vi "ScriptAccessorVIs.vi"(5 "Virtual Folder Name":string, 6 "Create as Properties":bool, 7 "Include error terminals":bool, 8 "error in (no error)":errorcluster, 9 "Make Class Terminals Dynamic":bool, 10 "Access":T1, 11 "BaseAccessorScripter in":refnum<class "BaseAccessorScripter.lvclass">) -> (0 "error out":errorcluster, 3 "BaseAccessorScripter out":refnum<class "BaseAccessorScripter.lvclass">)   [LabVIEW 2021, in "MemberVICreation.lvlib" / "BaseAccessorScripter.lvclass"]
uses:
  <resource>/Framework/Providers/LVClassLibrary/NewAccessors/BaseAccessorScripter/BaseAccessorScripter.lvclass
  <resource>/Framework/Providers/LVClassLibrary/NewAccessors/CLSUIP_Access.ctl
  <resource>/Framework/Providers/LVClassLibrary/NewAccessors/BaseAccessorScripter/BaseAccessorScripter.lvclass/BaseAccessorScripter.ctl
  <resource>/Framework/Providers/LVClassLibrary/NewAccessors/MemberVICreation.lvlib
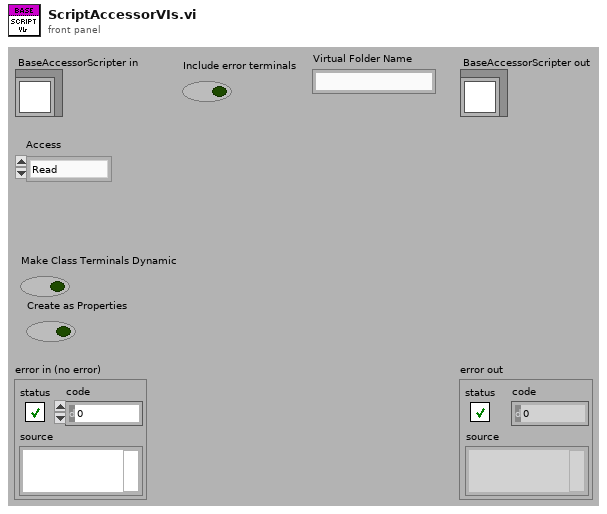
[diagram p1: front panel]
types:
  T1 = typedef "MemberVICreation.lvlib/CLSUIP_Access.ctl" = enum16{"Read", "Write", "R/W"}
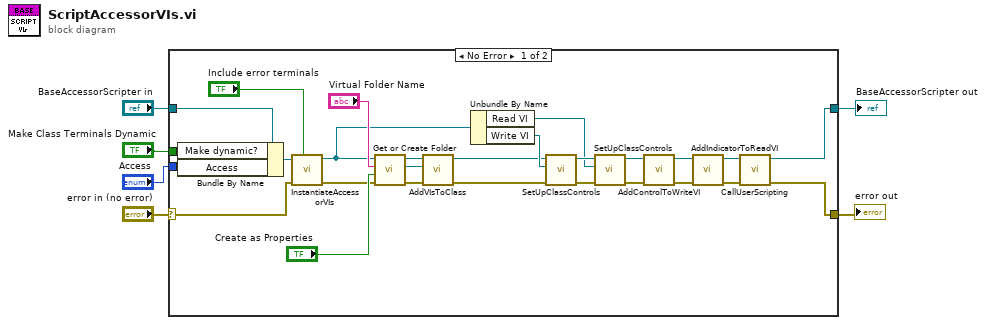
[diagram p0: block diagram]
diagram:
  n1 = case shown="No Error" "error in (no error)" {
    selector: "error in (no error)" -> [w29 w35]
    tunnel: [w19 w35] -> w5
    tunnel: [w18 w34] -> w3
    tunnel: "BaseAccessorScripter in" -> [w33 w34]
    tunnel: "Make Class Terminals Dynamic" -> [w32 _]
    tunnel: "Access" -> [w31 _]
    frame No Error {
      n2 = Bundle By Name(cluster=w33, "Make dynamic?"=w32, "Access"=w31) -> (w30:refnum<class "BaseAccessorScripter.lvclass">)
      n3 = call <resource>:"InstantiateAccessorVIs.vi"("Include error terminals"="Include error terminals", "error in (no error)"=w29, "BaseAccessorScripter in"=w30) -> ("error out"=w10:errorcluster, "BaseAccessorScripter out"=w7:refnum<class "BaseAccessorScripter.lvclass">)  [unwired: 7 out]
      n4 = call-dynamic "Get or Create Folder.vi"("error in (no error)"=w10, "CreateAsProperties"="Create as Properties", "Virtual Folder Name"="Virtual Folder Name", "BaseAccessorScripter in"=w7) -> ("error out"=w14:errorcluster, "Folder Refnum out"=w13:refnum<vi>, "BaseAccessorScripter out"=w17:refnum<class "BaseAccessorScripter.lvclass">)  [unwired: 5 in]
      n5 = call <resource>:"AddVIsToClass.vi"("error in (no error)"=w14, "Destination Folder"=w13, "BaseAccessorScripter in"=w17) -> ("error out"=w9:errorcluster, "BaseAccessorScripter out"=w8:refnum<class "BaseAccessorScripter.lvclass">)  [unwired: 7 in]
      n6 = Unbundle By Name(w7) -> ("Read VI"=w25:refnum<vi>, "Write VI"=w26:refnum<vi>)
      n7 = call <resource>:"SetUpClassControls.vi"("error in (no error)"=w9, "VI Reference"=w26, "Scripter Class"=w8) -> ("error out"=w27:errorcluster, "Scripter Class out"=w28:refnum<class "BaseAccessorScripter.lvclass">)  [unwired: 7 out]
      n8 = call <resource>:"SetUpClassControls.vi"("error in (no error)"=w27, "VI Reference"=w25, "Scripter Class"=w28) -> ("error out"=w23:errorcluster, "Scripter Class out"=w24:refnum<class "BaseAccessorScripter.lvclass">)  [unwired: 7 out]
      n9 = call <resource>:"AddControlToWriteVI.vi"("error in (no error)"=w23, "BaseAccessorScripter in"=w24) -> ("error out"=w21:errorcluster, "BaseAccessorScripter out"=w22:refnum<class "BaseAccessorScripter.lvclass">)  [unwired: 8 out]
      n10 = call <resource>:"AddIndicatorToReadVI.vi"("error in (no error)"=w21, "BaseAccessorScripter in"=w22) -> ("error out"=w12:errorcluster, "BaseAccessorScripter out"=w11:refnum<class "BaseAccessorScripter.lvclass">)  [unwired: 8 out]
      n11 = call-dynamic "CallUserScripting.vi"("error in"=w12, "BaseAccessorScripter in"=w11) -> ("error out"=w19:errorcluster, "BaseAccessorScripter out"=w18:refnum<class "BaseAccessorScripter.lvclass">)  [unwired: 8 in]
    }
    frame Error {
    }
  }
  "error out" <- w5
  "BaseAccessorScripter out" <- w3
